vi "Control_Snake.vi"(8 "Player":T1) -> ()   [LabVIEW 2018]
uses:
  TypDefs/Player_Enum.ctl
  TypDefs/Direction_Enum.ctl
  <vilib>/rvi/Emulation/niFpgaGetClockAttributes.vi
  <vilib>/rvi/Emulation/niFpgaSctlEmulationGetInTimedLoop.vi
  <vilib>/rvi/Emulation/niFpgaEmulationReportErrorSimple.vi
  <vilib>/rvi/Emulation/niFpgaProcessEmulError.vi
  Global_GameOver.vi
  Game/Global_ScorePlayer1.vi
  Game/Global_ScorePlayer2.vi
  <vilib>/rvi/Emulation/niFpgaCriticalErrorInLSC.vi
panel:
  out "JoystickLatch":bool
  out "JoystickRight":bool
  out "JoystickLeft":bool
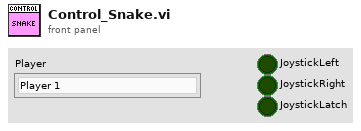
[diagram p1: front panel]
types:
  T1 = typedef "Player_Enum.ctl" = enum16{"Player 1", "Player 2"}
  T2 = typedef "Direction_Enum.ctl" = enum8{"Left", "Right", "Up", "Down"}
  T3 = typedef "Tile_Enum.ctl" = enum8{"Empty", "Snake1_HeadPointingUp", "Snake1_HeadPointingDown", "Snake1_HeadPointingLeft", "Snake1_HeadPointingRight", "Snake1_DeadPointingUp", "Snake1_DeadPointingDown", "Snake1_DeadPointingLeft", "Snake1_DeadPointingRight", "Snake1_TailPointingUp", "Snake1_TailPointingDown", "Snake1_TailPointingLeft", "Snake1_TailPointingRight", "Snake1_Horizontal", "Snake1_Vertical", "Snake1_UpperLeftCorner", "Snake1_UpperRightCorner", "Snake1_LowerLeftCorner", "Snake1_LowerRightCorner", "Snake2_HeadPointingUp", "Snake2_HeadPointingDown", "Snake2_HeadPointingLeft", "Snake2_HeadPointingRight", "Snake2_DeadPointingUp", "Snake2_DeadPointingDown", "Snake2_DeadPointingLeft", "Snake2_DeadPointingRight", "Snake2_TailPointingUp", "Snake2_TailPointingDown", "Snake2_TailPointingLeft", "Snake2_TailPointingRight", "Snake2_Horizontal", "Snake2_Vertical", "Snake2_UpperLeftCorner", "Snake2_UpperRightCorner", "Snake2_LowerLeftCorner", "Snake2_LowerRightCorner", "Wall_Horizontal", "Wall_Vertical", "Wall_UpperLeftCorner", "Wall_UpperRightCorner", "Wall_LowerLeftCorner", "Wall_LowerRightCorner", "Pickup_SpeedUp", "Pickup_Stop", "Pickup_Item1", "Pickup_Item2", "Pickup_Item3", "Pickup_Item4", "Pickup_Item5", "Pickup_Item6"}
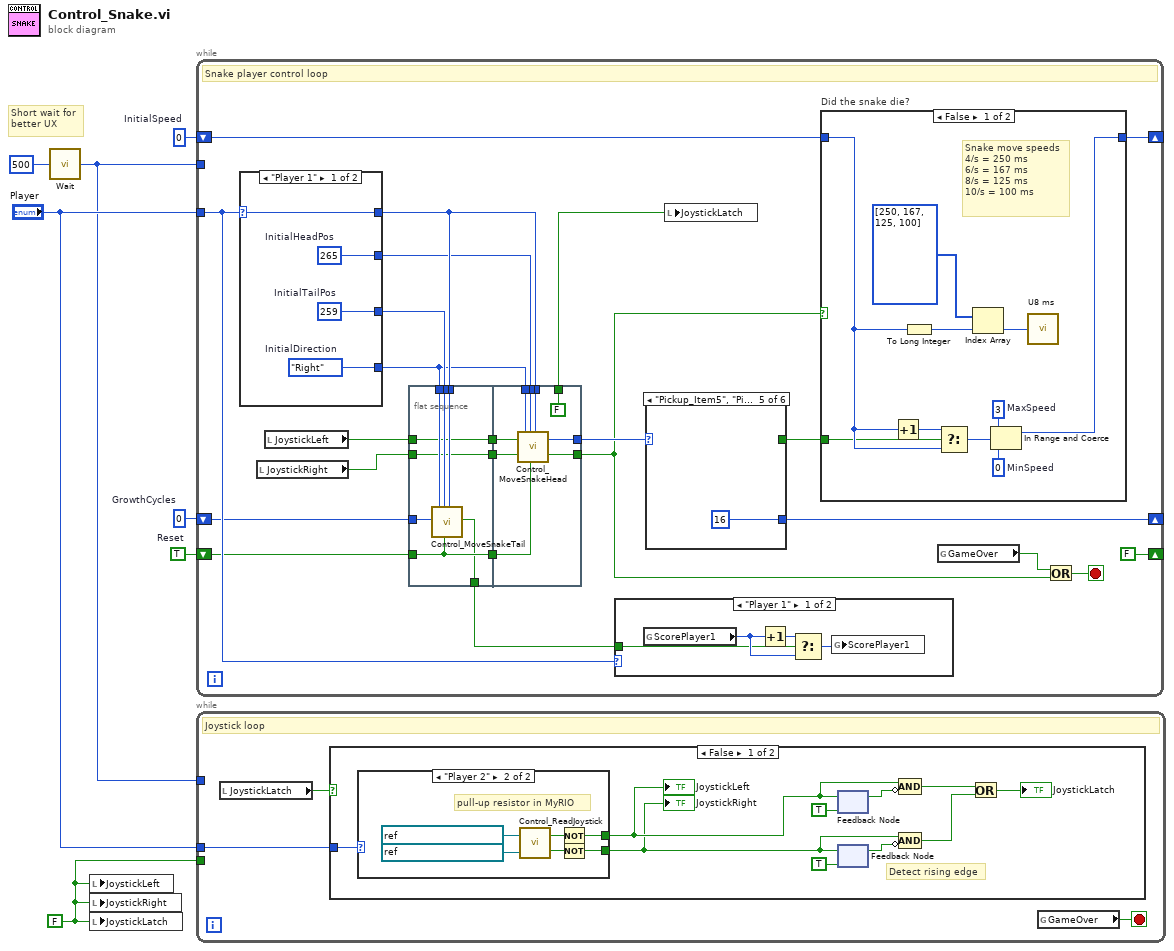
[diagram p0: block diagram]
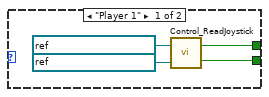
[diagram p2: hidden frame]
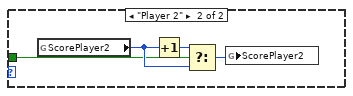
[diagram p4: hidden frame]
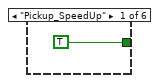
[diagram p5: hidden frame]
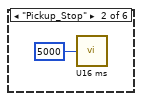
[diagram p6: hidden frame]
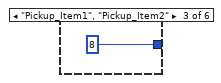
[diagram p7: hidden frame]
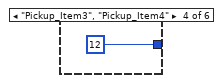
[diagram p8: hidden frame]
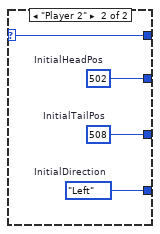
[diagram p10: hidden frame]
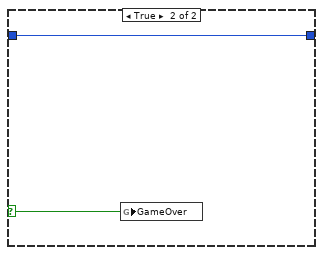
[diagram p11: hidden frame]
diagram:
  w3 = FALSE ("JoystickLeft")
  w4 = i8 0  # GrowthCycles
  w5 = i16 0  # InitialSpeed
  w6 = TRUE  # Reset
  # "Short wait for\nbetter UX"
  n1 = call "Wait"("Count(mSec)"=u16 500) -> ("Tick Count(mSec)"=w1:u16)
  n2 = local write "JoystickLeft"(w3) -> ()
  n3 = local write "JoystickRight"(w3) -> ()
  n4 = local write "JoystickLatch"(w3) -> ()
  n5 = while {
    tunnel: "Player" -> [w30]
    shift-right: [FALSE ("Reset")] -> _
    shift-left: w6 -> [w17]
    shift-right: [w24] -> _
    shift-left: w5 -> [w25]
    shift-right: [w29] -> _
    shift-left: w4 -> [w21]
    tunnel: w1 -> [_]
    stop <- w28 stop-if-true
    # "Snake player control loop"
    n6 = case shown="\"Player 1\"" w30 {
      selector: w30 -> [w64 w68]
      tunnel: [w64 w68] -> w14
      tunnel: [w63 w67] -> w13
      tunnel: [w62 w66] -> w12
      tunnel: [w61 w65] -> w23
      frame "Player 1" {
        w61 = i16 259  # InitialTailPos
        w63 = i16 265  # InitialHeadPos
        w62 = Direction_Enum."Right"  # InitialDirection
      }
      frame "Player 2" {
        w65 = i16 508  # InitialTailPos
        w67 = i16 502  # InitialHeadPos
        w66 = Direction_Enum."Left"  # InitialDirection
      }
    }
    n7 = local read "JoystickRight"() -> (w9:bool)
    n8 = local read "JoystickLeft"() -> (w10:bool)
    n9 = flat-sequence {
      tunnel: w14 -> [w44]
      tunnel: w23 -> [w45]
      tunnel: w21 -> [w43]
      tunnel: [w42] -> w19
      tunnel: w10 -> [w42]
      tunnel: [w41] -> w18
      tunnel: w9 -> [w41]
      tunnel: w17 -> [w40]
      tunnel: [w40] -> w16
      tunnel: w12 -> [w46]
      tunnel: [w39] -> w8
      tunnel: [w55] -> w15
      tunnel: [w54] -> w20
      tunnel: w19 -> [w53]
      tunnel: w18 -> [w52]
      tunnel: w14 -> [w51]
      tunnel: w13 -> [w50]
      tunnel: w12 -> [w49]
      tunnel: w16 -> [w48]
      tunnel: [FALSE ("JoystickLatch")] -> w11
      frame #0 {
        n10 = call "Control_MoveSnakeTail.vi"("AddGrowthCycles"=w43, "InitialDirection"=w46, "InitialPosition"=w45, "Reset"=w40, "Player"=w44) -> ("Growing?"=w39:bool)  [unwired: 14 in]
      }
      frame #1 {
        n11 = call "Control_MoveSnakeHead.vi"("InputLeft"=w53, "InputRight"=w52, "InitialDirection"=w49, "InitialPosition"=w50, "Reset"=w48, "Player"=w51) -> ("PickUp"=w54:T3, "PlayerDied?"=w55:bool)  [unwired: 12 in]
      }
    }
    n12 = case shown="\"Player 1\"" w30 {
      tunnel: w8 -> [w31 w35]
      frame "Player 1" {
        n13 = global read "Global_ScorePlayer1.vi" "ScorePlayer1"() -> (w34:u16)
        n14 = Increment(x=w34) -> (x+1=w33:u16)
        n15 = Select(t=w33, s=w31, f=w34) -> (s? t:f=w32:u16)
        n16 = global write "Global_ScorePlayer1.vi" "ScorePlayer1"(w32) -> ()
      }
      frame "Player 2" {
        n17 = global read "Global_ScorePlayer2.vi" "ScorePlayer2"() -> (w38:u16)
        n18 = Increment(x=w38) -> (x+1=w37:u16)
        n19 = Select(t=w37, s=w35, f=w38) -> (s? t:f=w36:u16)
        n20 = global write "Global_ScorePlayer2.vi" "ScorePlayer2"(w36) -> ()
      }
    }
    n21 = case shown="\"Pickup_Item5\", \"Pickup_Item6\"" w20 {
      tunnel: [_ _ i8 8 i8 12 i8 16 _] -> w29
      tunnel: [TRUE _ _ _ _ _] -> w22
      frame "Pickup_SpeedUp" {
      }
      frame "Pickup_Stop" {
        n22 = call "U16 ms"("Count(mSec)"=u16 5000) -> ()  [unwired: 1 out]
      }
      frame "Pickup_Item1", "Pickup_Item2" {
      }
      frame "Pickup_Item3", "Pickup_Item4" {
      }
      frame "Pickup_Item5", "Pickup_Item6" {
      }
      frame Default {
      }
    }
    n23 = local write "JoystickLatch"(w11) -> ()
    n24 = case "Did the snake die?" shown="False" w15 {
      selector: w15 -> [_ w79]
      tunnel: w25 -> [w71 w80]
      tunnel: [w76 w80] -> w24
      tunnel: w22 -> [w69 _]
      frame False {
        w77 = i16 3  # MaxSpeed
        w78 = i16 0  # MinSpeed
        # "Snake move speeds\n4/s = 250 ms\n6/s = 167 ms\n8/s = 125 ms\n10/s = 100 ms"
        n25 = Increment(x=w71) -> (x+1=w70:i16)
        n26 = To Long Integer(number=w71) -> (32bit integer=w74:i32)
        n27 = Select(t=w70, s=w69, f=w71) -> (s? t:f=w72:i16)
        n28 = Index Array(array=u8[] [250, 167, 125, 100], index=w74) -> (element=w75:u8)
        n29 = In Range and Coerce(upper limit=w77, x=w72, lower limit=w78) -> (coerced(x)=w76:i16)  [unwired: 1 out]
        n30 = call "U8 ms"("Count(mSec)"=w75) -> ()  [unwired: 1 out]
      }
      frame True {
        n31 = global write "Global_GameOver.vi" "GameOver"(w79) -> ()
      }
    }
    n32 = global read "Global_GameOver.vi" "GameOver"() -> (w27:bool)
    n33 = Or(x=w27, y=w15) -> (x .or. y?=w28:bool)
  }
  n34 = while {
    tunnel: "Player" -> [w82]
    tunnel: w3 -> [_]
    tunnel: w1 -> [_]
    stop <- w83 stop-if-true
    # "Joystick loop"
    n35 = local read "JoystickLatch"() -> (w81:bool)
    n36 = case shown="False" w81 {
      tunnel: w82 -> [w93 _]
      frame False {
        # "Detect rising edge"
        n37 = case shown="\"Player 2\"" w93 {
          tunnel: [w97 w99] -> w86
          tunnel: [w96 w98] -> w85
          frame "Player 1" {
            n38 = call "Control_ReadJoystick.vi"("joy_left [FPGA DI]"=refnum<k21> "ConnectorC/DIO6", "joy_right [FPGA DI]"=refnum<k21> "ConnectorC/DIO7") -> ("Left"=w97:bool, "Right"=w96:bool)  [unwired: 16 in]
          }
          frame "Player 2" {
            # "pull-up resistor in MyRIO"
            n39 = call "Control_ReadJoystick.vi"("joy_left [FPGA DI]"=refnum<k21> "ConnectorB/DIO0", "joy_right [FPGA DI]"=refnum<k21> "ConnectorB/DIO1") -> ("Left"=w103:bool, "Right"=w102:bool)  [unwired: 16 in]
            n40 = Not(x=w103) -> (.not. x?=w99:bool)
            n41 = Not(x=w102) -> (.not. x?=w98:bool)
          }
        }
        "JoystickRight" <- w85
        "JoystickLeft" <- w86
        n42 = feedback #1(TRUE) -> (w91:bool)
        n43 = feedback-in #1(w86) -> ()
        n44 = feedback #2(TRUE) -> (w90:bool)
        n45 = feedback-in #2(w85) -> ()
        n46 = Compound Arithmetic op=AND(w86, invert w91) -> (w88:bool)
        n47 = Compound Arithmetic op=AND(w85, invert w90) -> (w87:bool)
        n48 = Or(x=w88, y=w87) -> (x .or. y?=→"JoystickLatch":bool)
      }
      frame True {
        # "Iqnore joystick input until the snake has moved"
      }
    }
    n49 = global read "Global_GameOver.vi" "GameOver"() -> (w83:bool)
  }
